vi "AttrGetAssemblyVersion.vi"(8 "error in":errorcluster, 11 "MCanHandleIn":T1) -> (0 "error out":errorcluster, 2 "Value":string, 3 "MCanHandleOut":T1)   [LabVIEW 2011, in "Konvolucio MCAN120803.lvlib"]
doc: "The Konvolucio.MCAN120803.dll Assembly Version."
uses:
  <instrlib>/Konvolucio MCAN120803/Konvolucio MCAN120803.lvlib
  <instrlib>/Konvolucio MCAN120803/Types/CanHandleType.ctl
  C:/Program Files/National Instruments/LabVIEW 2011/instr.lib/Konvolucio MCAN120803/Private/Konvolucio.MCAN120803.API.dll
  Private/Konvolucio.MCAN120803.API.dll
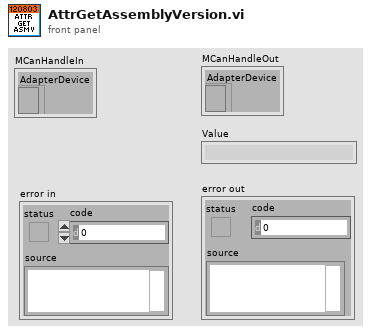
[diagram p1: front panel]
types:
  T1 = typedef "Konvolucio MCAN120803.lvlib/CanHandleType.ctl" = cluster{"AdapterDevice":refnum<k24>}
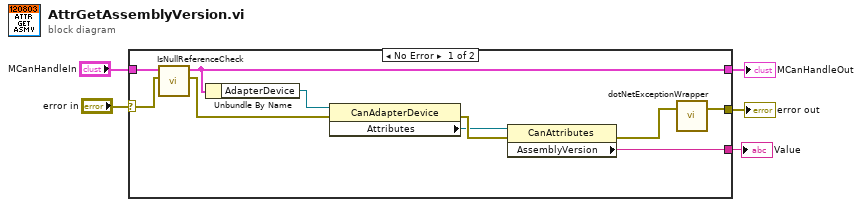
[diagram p0: block diagram]
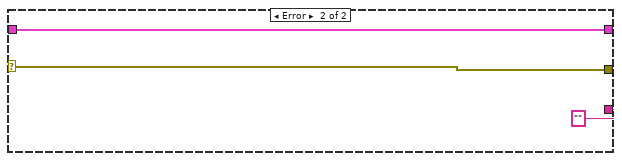
[diagram p2: hidden frame]
diagram:
  n1 = case shown="No Error" "error in" {
    selector: "error in" -> [w9 w18]
    tunnel: [w15 w18] -> w5
    tunnel: "MCanHandleIn" -> [w14 w17]
    tunnel: [w13 w17] -> w2
    tunnel: [w11 "" ("Attributes.FirmwareRev")] -> w1
    frame No Error {
      n2 = call <instrlib>:"IsNullReferenceCheck.vi"("error in"=w9, "MCanHandleIn"=w14) -> ("error out"=w8:errorcluster, "MCanHandleOut"=w13:T1)  [unwired: 5 in]
      n3 = Unbundle By Name(w13) -> ("AdapterDevice"=w10:refnum<k24>)
      n4 = property class="CanAdapterDevice"(reference=w10, error in=w8) -> (error out=w7:errorcluster, "Attributes"=w6:refnum<k24>)  [unwired: 1 out]
      n5 = property class="CanAttributes"(reference=w6, error in=w7) -> (error out=w12:errorcluster, "AssemblyVersion"=w11:string)  [unwired: 1 out]
      n6 = call <instrlib>:"dotNetExceptionWrapper.vi"("error in"=w12) -> ("error out"=w15:errorcluster)  [unwired: 2 in]
    }
    frame Error {
    }
  }
  "error out" <- w5
  "MCanHandleOut" <- w2
  "Value" <- w1
